vi "SetLocal.vi"(8 "Error In":errorcluster, 11 "Keithley 2602 In":refnum<visa-resource-name>) -> (0 "Error Out":errorcluster, 3 "Keithley 2602 Out":refnum<visa-resource-name>)   [LabVIEW 2013, in "Keithley-2602.lvlib"]
uses:
  Keithley-2602.lvlib
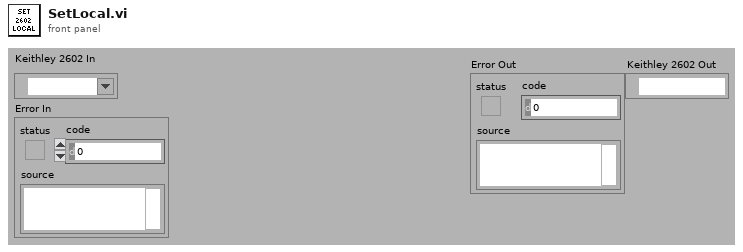
[diagram p1: front panel]
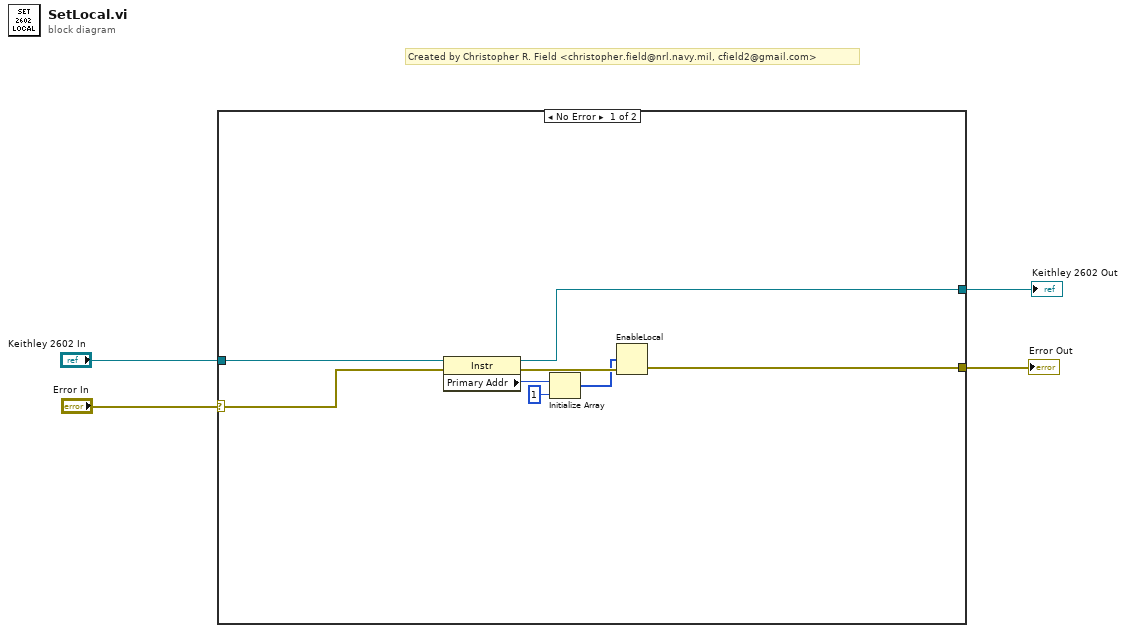
[diagram p0: block diagram]
diagram:
  # "Created by Christopher R. Field <christopher.field@nrl.navy.mil, cfield2@gmail.com>"
  n1 = case shown="No Error" "Error In" {
    selector: "Error In" -> [w5 w13]
    tunnel: "Keithley 2602 In" -> [w8 w14]
    tunnel: [w7 w13] -> w3
    tunnel: [w6 w14] -> w2
    frame No Error {
      n2 = property class="Instr"(reference=w8, error in=w5) -> (reference out=w6:refnum<visa-resource-name>, error out=w10:errorcluster, "Primary Addr"=w12:u16)
      n3 = Initialize Array(w12, u8 1 ("dimension size")) -> (w9:u16[])
      n4 = EnableLocal(2:w10, 3:w9) -> (0:w7:errorcluster)  [unwired: 1 in, 1 out]
    }
    frame Error {
    }
  }
  "Error Out" <- w3
  "Keithley 2602 Out" <- w2
